vi "FP_Set Random Position.vi"(8 "Error":errorcluster, 9 "Border":i16=100, 11 "Vi Ref (this Vi)":refnum<vi>) -> (0 "Error Out":errorcluster, 3 "Vi Ref (this Vi) Out":refnum<vi>, 5 "Final Rect Out":T1, 7 "Primary Workspace Out":T1)   [LabVIEW 2020]
uses:
  <vilib>/Utility/miscctls.llb/LVRectTypeDef.ctl
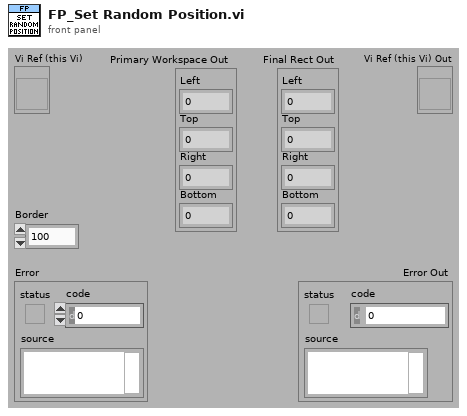
[diagram p1: front panel]
types:
  T1 = typedef "LVRectTypeDef.ctl" = cluster{"Left":i16, "Top":i16, "Right":i16, "Bottom":i16}
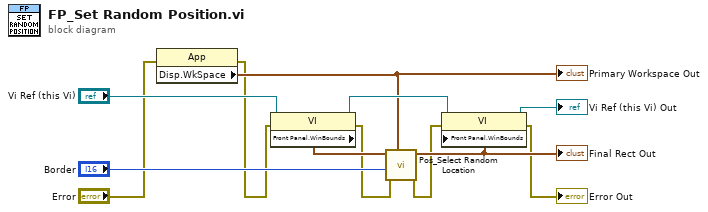
[diagram p0: block diagram]
diagram:
  n1 = property class="App"(error in="Error") -> (error out=w2:errorcluster, "Disp.WkSpace"=w4:T1)  [unwired: 1 in, 1 out]
  "Primary Workspace Out" <- w4
  n2 = property class="VI"(reference="Vi Ref (this Vi)", error in=w2) -> (reference out=w11:refnum<vi>, error out=w7:errorcluster, "Front Panel.WinBounds"=w9:T1)
  n3 = call "Pos_Select Random Location.vi"("Work Space"=w4, "Error"=w7, "Min Border"="Border", "Window Bounds"=w9) -> ("Error Out"=w6:errorcluster, "Window Bounds Out"=w8:T1)  [unwired: 6 in]
  "Final Rect Out" <- w8
  n4 = property class="VI"(reference=w11, error in=w6, "Front Panel.WinBounds"=w8) -> (reference out=→"Vi Ref (this Vi) Out":refnum<vi>, error out=→"Error Out":errorcluster)
